vi "UUID.vi"() -> (0 "UUID":string)   [LabVIEW 2016, in "EPUB.lvclass"]
uses:
  EPUB.lvclass
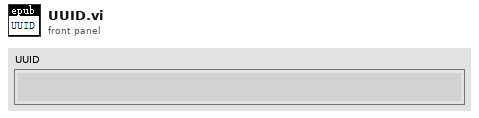
[diagram p1: front panel]
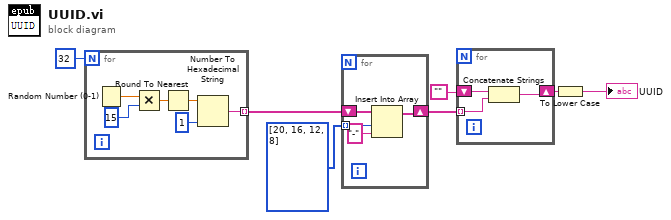
[diagram p0: block diagram]
diagram:
  n1 = for {
    N: 32 -> [_]
    tunnel: [w9] -> w6 mode=indexing
    n2 = Random Number (0-1)() -> (number: 0 to 1=w13:dbl)
    n3 = Multiply(x=w13, y=u32 15) -> (x*y=w11:dbl)
    n4 = Round To Nearest(number=w11) -> (nearest integer value=w10:dbl)
    n5 = Number To Hexadecimal String(1:i16 1 ("宽度(-)"), 2:w10) -> (0:w9:string)
  }
  n6 = for {
    shift-right: [w16] -> w4
    shift-left: w6 -> [w17]
    tunnel: i32[] [20, 16, 12, 8] -> [w15] mode=indexing
    n7 = Insert Into Array(array=w17, index=w15, new element="-" ("新元素/子数组")) -> (w16:string[])
  }
  n8 = for {
    tunnel: w4 -> [w19] mode=indexing
    shift-right: [w18] -> w2
    shift-left: "" -> [w20]
    n9 = Concatenate Strings(w20, w19) -> (w18:string)
  }
  n10 = To Lower Case(string=w2) -> (all lower case string=→"UUID":string)
